vi "reward_behavior_michelle_visjitter_conswin.vi"() -> ()   [LabVIEW 2019]
doc: "The myRIO Project template acquires acceleration data from the onboard accelerometer and displays the changes of acceleration values in a waveform chart."
uses:
  <vilib>/Analysis/Matrix/Datatypes/RealMatrix.ctl
  <vilib>/myRIO/Common/Instrument Driver Framework/myRIO v1.0/Encoder/typedefs/Encoder Signal Mode.ctl
  <vilib>/myRIO/Instrument Drivers/Onboard IO/Encoder/typedefs/Encoder Reference.ctl
  <vilib>/myRIO/Common/Instrument Driver Framework/Utilities/typedefs/myRIO Generic Hardware Reference.ctl
  <vilib>/myRIO/Common/Instrument Driver Framework/Utilities/typedefs/Hardware Version Enum.ctl
  <vilib>/myRIO/Common/Instrument Driver Framework/Utilities/typedefs/myRIO v1.0 Reference.ctl
  <vilib>/myRIO/Common/Instrument Driver Framework/Utilities/typedefs/Generic FPGA Reference.ctl
  <vilib>/myRIO/Common/Instrument Driver Framework/myRIO v1.0/Encoder/typedefs/Encoder Channels Enum.ctl
  <vilib>/myRIO/Common/Instrument Driver Framework/myRIO v1.0/Encoder/typedefs/Encoder Configuration v1.0.ctl
  <vilib>/userdefined/High Color/nirio_resource_hc.ctl
  <vilib>/myRIO/Instrument Drivers/Onboard IO/DIO/typedefs/DIO Reference.ctl
  <vilib>/myRIO/Common/Instrument Driver Framework/myRIO v1.0/DIO/typedefs/DIO Channels List.ctl
  <vilib>/myRIO/Common/Instrument Driver Framework/myRIO v1.0/DIO/typedefs/DIO Channels Enum.ctl
  <vilib>/myRIO/Common/Instrument Driver Framework/Utilities/vis/Is FPGA Ref Available.vi
  <vilib>/myRIO/Common/Instrument Driver Framework/myRIO v1.0/Encoder/vis/myRIO v1.1 Open Encoder.vi
  <vilib>/myRIO/Instrument Drivers/Onboard IO/Encoder/vis/Read.vi
  <vilib>/myRIO/Common/Instrument Driver Framework/myRIO v1.0/DIO/vis/myRIO v1.1 Open DIO.vi
  <vilib>/myRIO/Instrument Drivers/Onboard IO/DIO/vis/Write.vi
  <vilib>/myRIO/Instrument Drivers/Onboard IO/DIO/vis/Read.vi
  <vilib>/myRIO/Common/Instrument Driver Framework/Utilities/vis/Validate Channels.vi
  <vilib>/myRIO/Common/Instrument Driver Framework/myRIO v1.0/Encoder/vis/myRIO v1.0 Reserve Encoder.vi
  <vilib>/myRIO/Common/Instrument Driver Framework/myRIO v1.0/DIO/vis/myRIO v1.0 Reserve DIO.vi
  <vilib>/myRIO/Common/Instrument Driver Framework/myRIO v1.0/Encoder/vis/myRIO v1.0 Build MUX Configuration Encoder.vi
  <vilib>/myRIO/Common/Instrument Driver Framework/myRIO v1.0/Resource Manager/vis/myRIO v1.0 Reserve Channel List.vi
  <vilib>/myRIO/Common/Instrument Driver Framework/myRIO v1.0/DIO/vis/myRIO v1.0 Build MUX Configuration DIO.vi
  <vilib>/myRIO/Common/Instrument Driver Framework/myRIO v1.0/Resource Manager/vis/myRIO v1.0 Create Configuration List.vi
  <vilib>/myRIO/Common/Instrument Driver Framework/myRIO v1.0/Resource Manager/vis/myRIO v1.0 Reserve Channel.vi
  <vilib>/myRIO/Common/Instrument Driver Framework/myRIO v1.0/Resource Manager/vis/myRIO v1.0 Unreserve Channel.vi
  <vilib>/myRIO/Common/Instrument Driver Framework/myRIO v1.0/Resource Manager/vis/myRIO v1.0 Build Mutex Name.vi
  <vilib>/Utility/VariantDataType/GetNumericInfo.vi
  <vilib>/Utility/error.llb/Error Cluster From Error Code.vi
  <vilib>/myRIO/Common/Instrument Driver Framework/myRIO v1.0/myRIO v1.1 Open.vi
  <vilib>/myRIO/Common/Instrument Driver Framework/Utilities/vis/IO Manager.vi
  <vilib>/myRIO/Common/Instrument Driver Framework/Utilities/vis/Configuration Manager.vi
  <vilib>/myRIO/Common/Instrument Driver Framework/myRIO v1.0/Resource Manager/vis/myRIO v1.0 Configure IO.vi
  <vilib>/myRIO/Common/Instrument Driver Framework/myRIO v1.0/myRIO v1.0 Close.vi
  <vilib>/myRIO/Common/Instrument Driver Framework/myRIO v1.0/Encoder/vis/myRIO v1.0 Configure Encoder.vi
  <vilib>/myRIO/Common/Instrument Driver Framework/myRIO v1.0/Encoder/vis/myRIO v1.0 Read Encoder.vi
  <vilib>/myRIO/Common/Instrument Driver Framework/myRIO v1.0/DIO/vis/myRIO v1.0 Read DIO.vi
  <vilib>/myRIO/Common/Instrument Driver Framework/myRIO v1.0/DIO/vis/myRIO v1.0 Write DIO.vi
  <vilib>/myRIO/Express VI/Onboard IO/Encoder/Encoder Express VI.xnode
  <vilib>/myRIO/Instrument Drivers/Onboard IO/Encoder/vis/myRIO Encoder Open.xnode
  <vilib>/myRIO/Express VI/Onboard IO/DI/DI Express VI.xnode
  <vilib>/myRIO/Instrument Drivers/Onboard IO/DIO/vis/myRIO DIO Open.xnode
  <vilib>/myRIO/Express VI/Onboard IO/DO/DO Express VI.xnode
  <vilib>/myRIO/Instrument Drivers/Onboard IO/Encoder/Encoder.lvlib
  <vilib>/myRIO/Instrument Drivers/Onboard IO/DIO/DIO.lvlib
  <vilib>/Analysis/Matrix/NI_Matrix.lvlib
panel:
  out "TimeOutDuration":i32
  out "ActiveTime":dbl
  out "ConsumptionGo":bool=TRUE
  out "Consumption_Period":i32
  out "Watch_Display":bool=TRUE
  in  "Give reward":bool
  out "Timings":dbl[](array[numeric])
  out "ISI":dbl
  out "ISI start time":dbl
  out "Time_out":bool=TRUE
  out "Time since lick":dbl
  out "Time of last lick":dbl
  out "Rewarded trials":dbl[](array[numeric])
  out "Rewards":u16
  out "Active Trial":bool
  out "Array temp2":T1
  out "Stimuli Loaded":bool
  out "Stim_ID":dbl[](array[numeric])
  out "Reward_mat":dbl[](array[numeric])
  out "Reward":bool=TRUE
  out "Frame clock":i32
  out "Licks":u32
  out "Lick":bool
  out "Time":dbl
  out "Stop":bool
  in  "Frames to collect":u32
  out "Overflow?":bool
  out "Counter Value":i32
  out "Velocity":dbl
  out "Velocity Plot":dbl[](graph)
  out "Velocity array":dbl[](array[numeric])
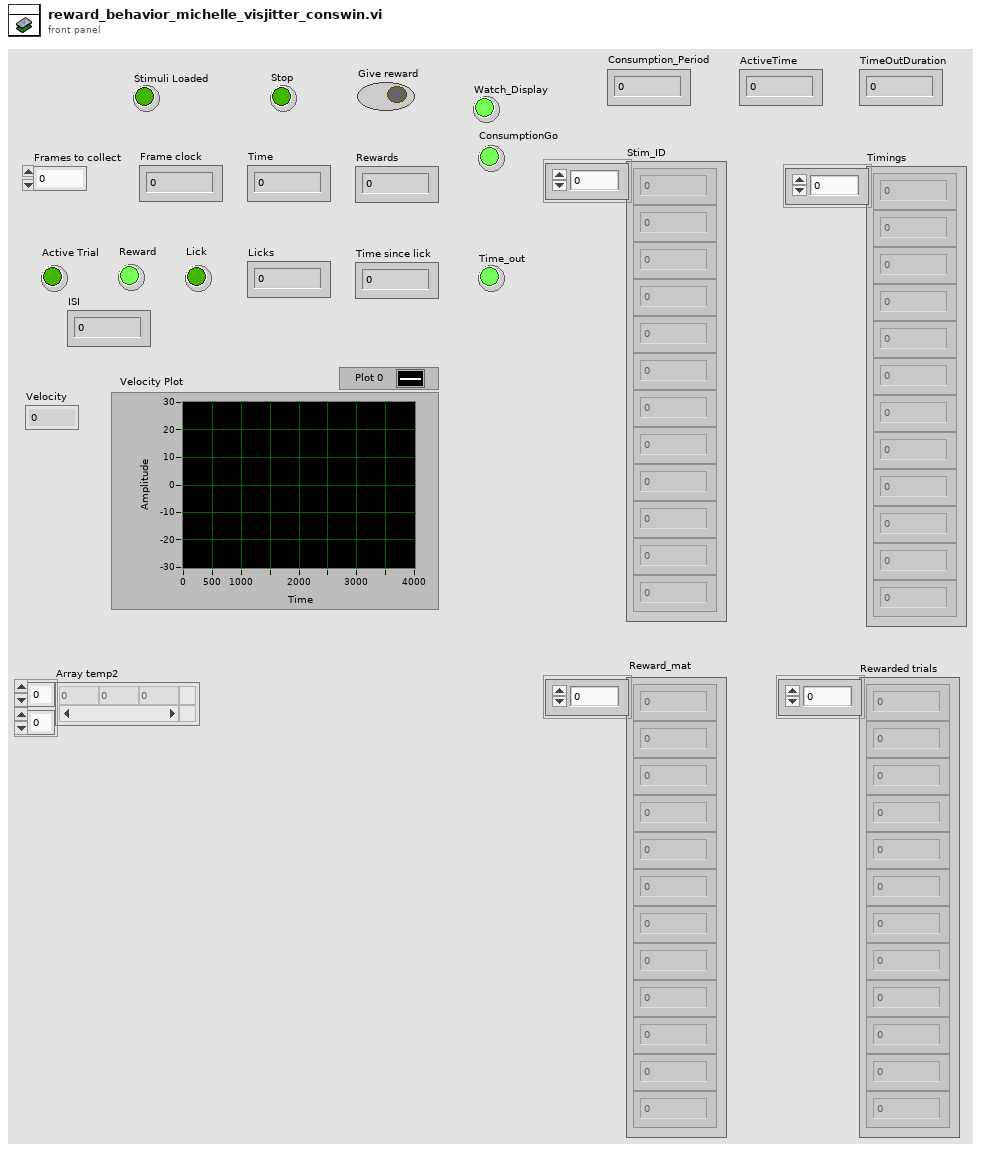
[diagram p1: front panel]
types:
  T1 = typedef "NI_Matrix.lvlib/RealMatrix.ctl" = dbl[][]
  T2 = typedef "Encoder.lvlib/Encoder Reference.ctl" = cluster{"myRIO Reference":T3, "Encoder Channels Enum":T7}
  T3 = typedef "myRIO Generic Hardware Reference.ctl" = cluster{"myRIO Model":T4, "myRIO Hardware Reference":T5}
  T4 = typedef "Hardware Version Enum.ctl" = enum16{"Unknown", "myRIO-1900", "myRIO-1950", "roboRIO", "NI ELVIS RIO CM", "ELVIS III"}
  T5 = typedef "myRIO v1.0 Reference.ctl" = cluster{"Generic FPGA Reference":T6, "Allow multiple opens":bool}
  T6 = typedef "Generic FPGA Reference.ctl" = refnum<k20>
  T7 = typedef "Encoder Channels Enum.ctl" = enum16{"Not Connected", "C/ENC0", "C/ENC1", "A/ENC", "A/ENC0", "A/ENC1", "A/ENC2", "A/ENC3", "A/ENC4", "A/ENC5", "A/ENC6", "A/ENC7", "A/ENC8", "A/ENC9", "B/ENC", "B/ENC0", "B/ENC1", "B/ENC2", "B/ENC3", "B/ENC4", "B/ENC5", "B/ENC6", "B/ENC7", "B/ENC8", "B/ENC9", "DIO/ENC0", "DIO/ENC1", "DIO/ENC2", "DIO/ENC3", "DIO/ENC4"}
  T8 = typedef "Encoder Signal Mode.ctl" = enum16{"Quadrature phase signal", "Step and direction signal"}
  T9 = typedef "nirio_resource_hc.ctl" = tag
  T10 = typedef "DIO.lvlib/DIO Reference.ctl" = cluster{"myRIO Reference":T3, "DIO Channels List":T11}
  T11 = typedef "DIO Channels List.ctl" = T12[]
  T12 = typedef "DIO Channels Enum.ctl" = enum16{"Not Connected", "C/DIO0", "C/DIO1", "C/DIO2", "C/DIO3", "C/DIO4", "C/DIO5", "C/DIO6", "C/DIO7", "A/DIO0", "A/DIO1", "A/DIO2", "A/DIO3", "A/DIO4", "A/DIO5", "A/DIO6", "A/DIO7", "A/DIO8", "A/DIO9", "A/DIO10", "A/DIO11", "A/DIO12", "A/DIO13", "A/DIO14", "A/DIO15", "A/DIO16", "A/DIO17", "A/DIO18", "A/DIO19", "B/DIO0", "B/DIO1", "B/DIO2", "B/DIO3", "B/DIO4", "B/DIO5", "B/DIO6", "B/DIO7", "B/DIO8", "B/DIO9", "B/DIO10", "B/DIO11", "B/DIO12", "B/DIO13", "B/DIO14", "B/DIO15", "B/DIO16", "B/DIO17", "B/DIO18", "B/DIO19", "LED0", "LED1", "LED2", "LED3", "Button0", "DIO/DIO0", "DIO/DIO1", "DIO/DIO2", "DIO/DIO3", "DIO/DIO4", "DIO/DIO5", "DIO/DIO6", "DIO/DIO7", "DIO/DIO8", "DIO/DIO9", "SPI/CS0", "SPI/CS1", "SPI/CS2", "SPI/CS3", "LED RADIO (Green)", "LED RADIO (Red)", "LED COMM (Green)", "LED COMM (Red)", "LED MODE (Green)", "LED MODE (Red)"}
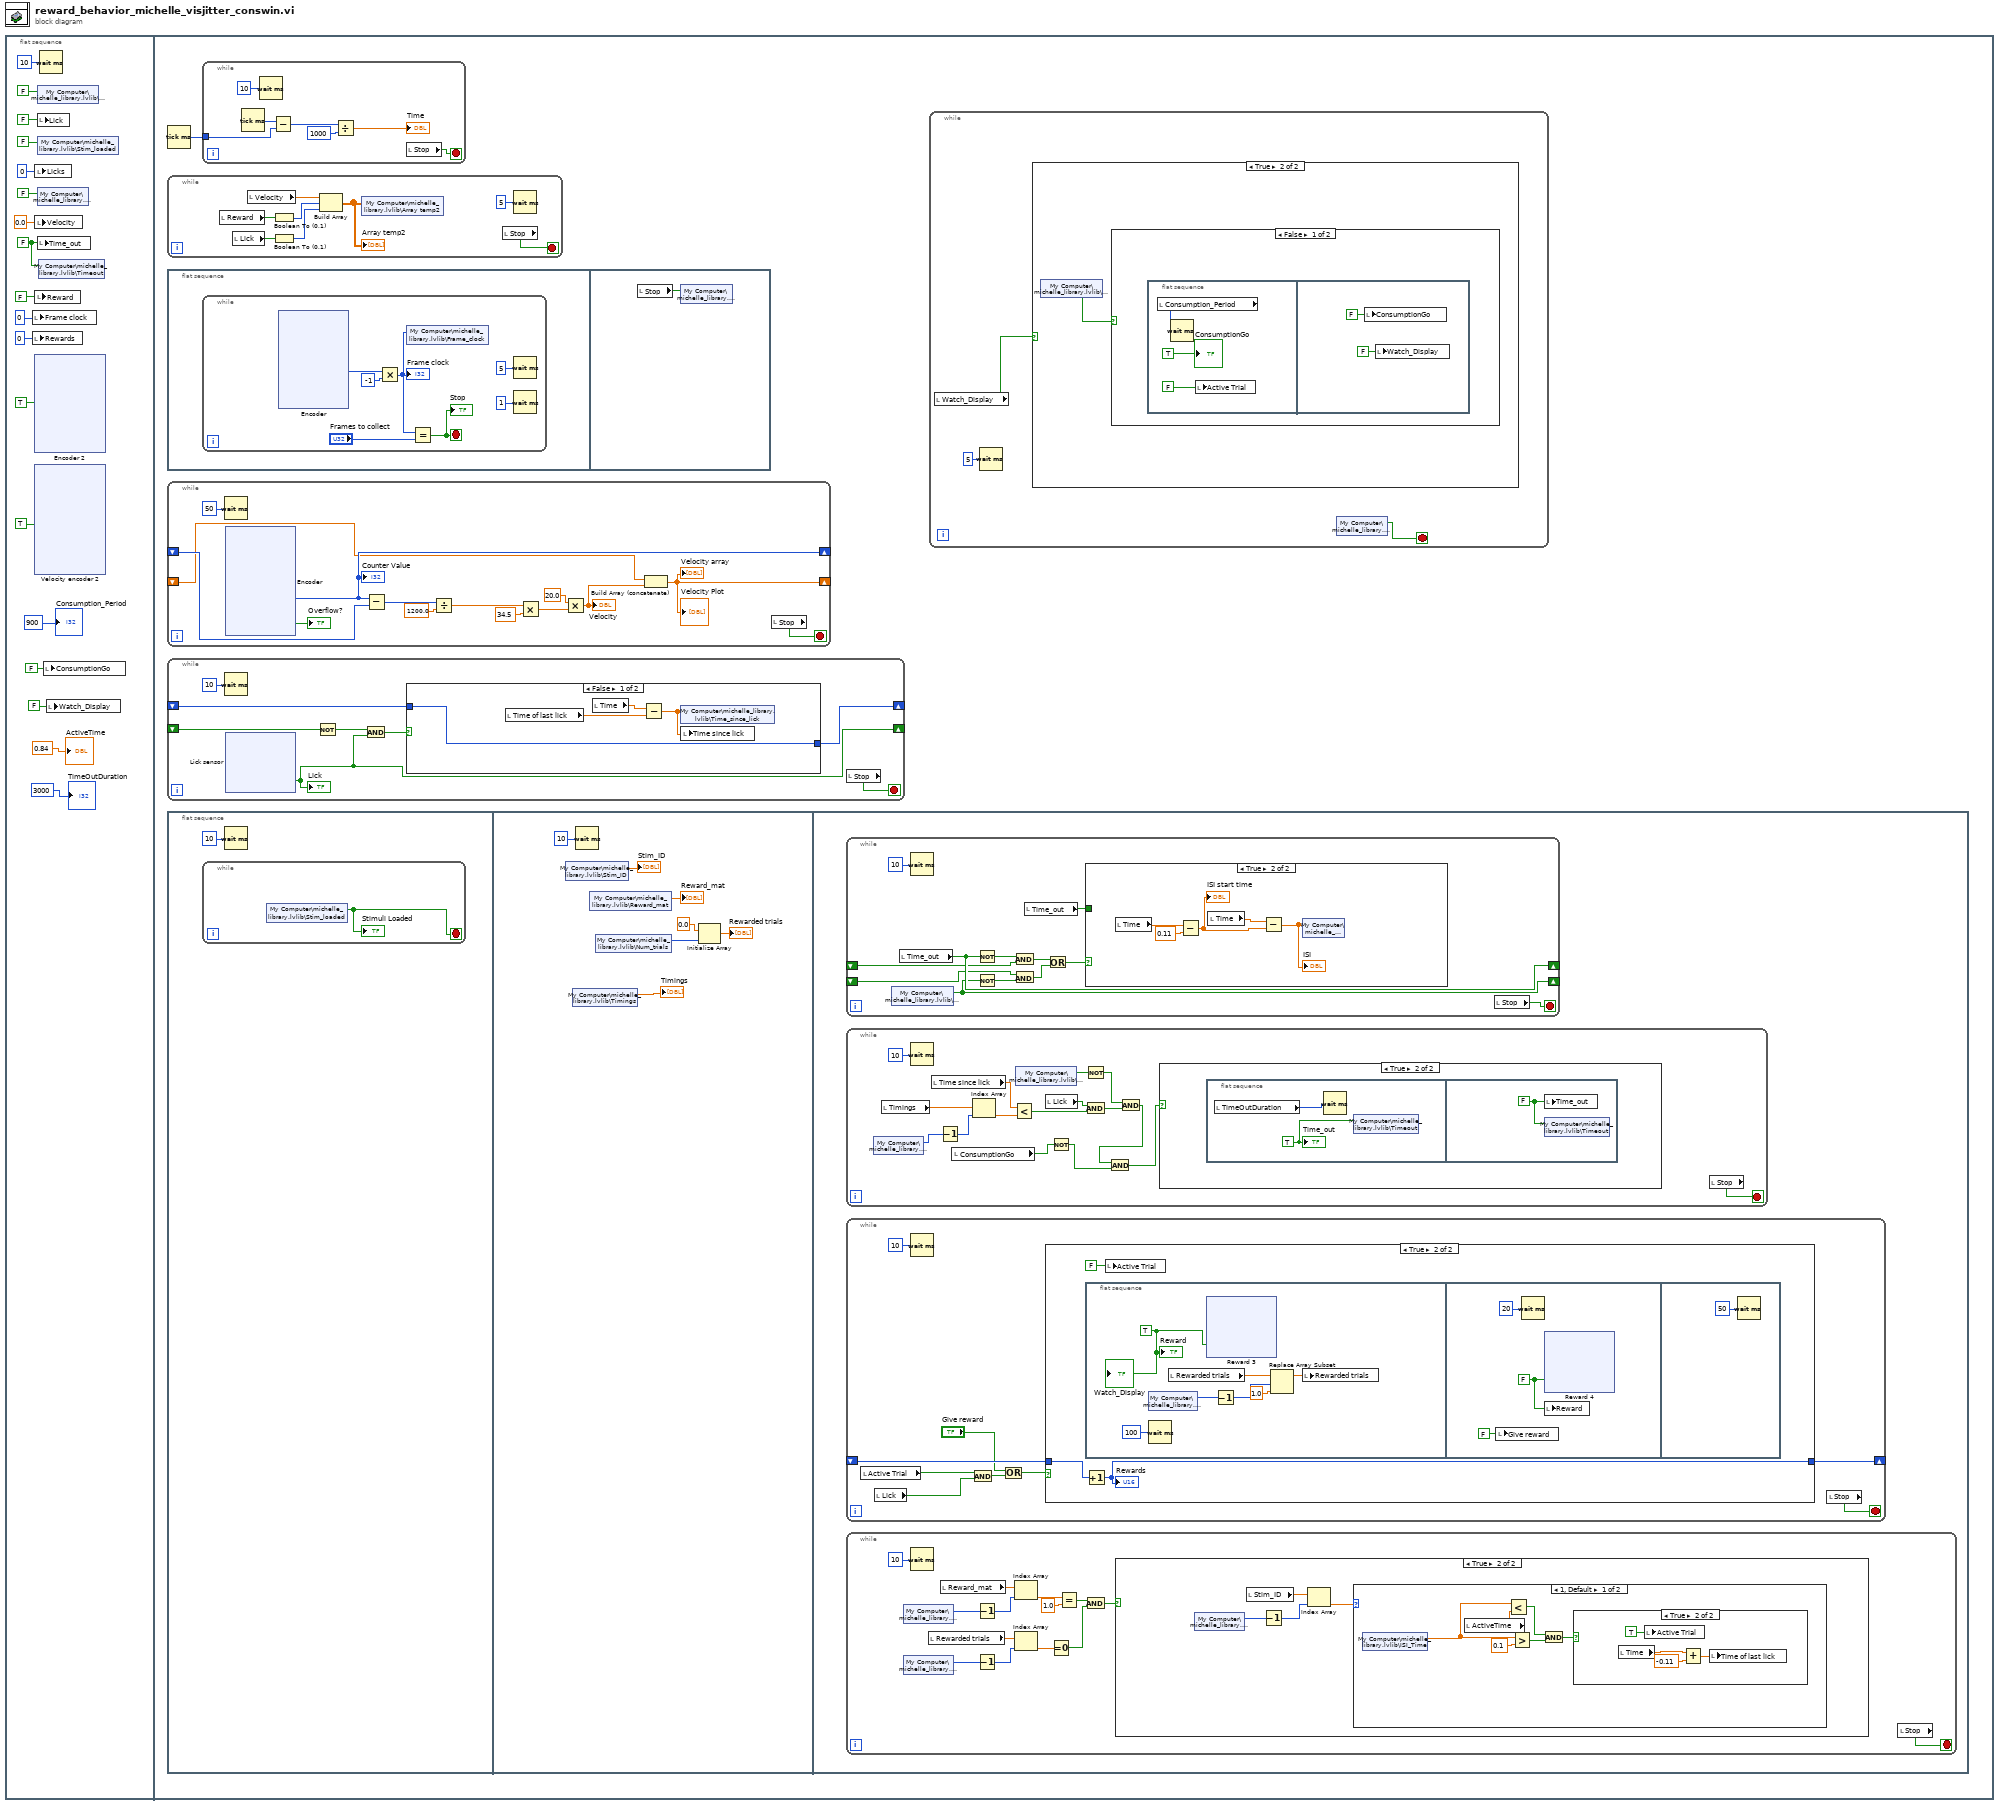
[diagram p0: block diagram]
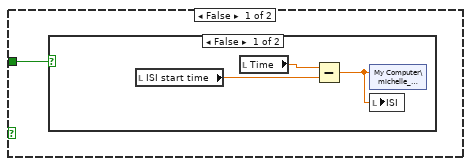
[diagram p5: hidden frame]
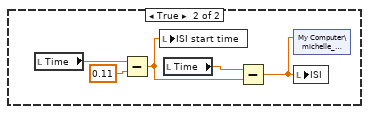
[diagram p6: hidden frame]
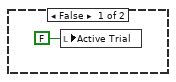
[diagram p7: hidden frame]
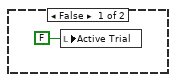
[diagram p8: hidden frame]
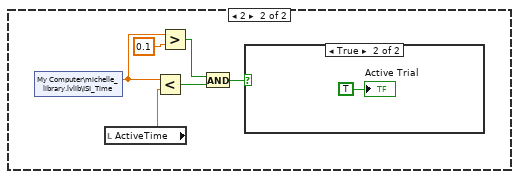
[diagram p9: hidden frame]
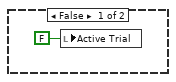
[diagram p10: hidden frame]
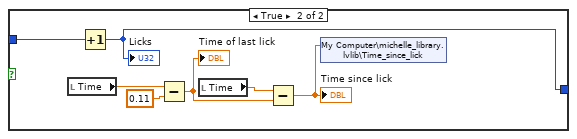
[diagram p12: hidden frame]
diagram:
  n1 = flat-sequence {
    frame #0 {
      w6 = FALSE ("Time_out")
      n2 = local write "Frame clock"(u32 0 ("Frames")) -> ()
      n3 = local write "Rewards"(u16 0 ("Rewards")) -> ()
      n4 = local write "Licks"(u32 0 ("Licks")) -> ()
      n5 = local write "Velocity"(0.0 ("Velocity")) -> ()
      n6 = local write "Reward"(FALSE ("Give reward")) -> ()
      n7 = xnode "Encoder 2"("Reset Counter"=TRUE) -> ()  [unwired: 1 in, 4 out]
      n8 = xnode "Velocity encoder 2"("Reset Counter"=TRUE) -> ()  [unwired: 1 in, 4 out]
      n9 = shared-variable "My Computer\\michelle_library.lvlib\\Display"(FALSE ("Display")) -> ()  [unwired: 1 in, 1 out]
      n10 = local write "Lick"(FALSE ("Lick")) -> ()
      n11 = shared-variable "My Computer\\michelle_library.lvlib\\Stim_loaded"(FALSE ("Stim_loaded")) -> ()  [unwired: 1 in, 1 out]
      n12 = shared-variable "My Computer\\michelle_library.lvlib\\Stop"(FALSE ("Stop")) -> ()  [unwired: 1 in, 1 out]
      n13 = local write "Time_out"(w6) -> ()
      n14 = shared-variable "My Computer\\michelle_library.lvlib\\Timeout"(w6) -> ()  [unwired: 1 in, 1 out]
      n15 = Wait (ms)(milliseconds to wait=u32 10) -> ()  [unwired: 1 out]
      n16 = local write "ConsumptionGo"(FALSE ("ConsumptionGo")) -> ()
      n17 = local write "Watch_Display"(FALSE ("Watch_Display")) -> ()
      "Consumption_Period" <- 900
      "ActiveTime" <- 0.84
      "TimeOutDuration" <- 3000
    }
    frame #1 {
      n18 = Tick Count (ms)() -> (millisecond timer value=w111:u32)
      n19 = while {
        stop <- w122 stop-if-true
        n20 = local read "Reward"() -> (w127:bool)
        n21 = local read "Lick"() -> (w128:bool)
        n22 = local read "Velocity"() -> (w126:dbl)
        n23 = Boolean To (0,1)(Boolean=w127) -> (0, 1=w125:i16)
        n24 = Boolean To (0,1)(Boolean=w128) -> (0, 1=w124:i16)
        n25 = Build Array(w126, w125, w124) -> (w121:T1)
        "Array temp2" <- w121
        n26 = shared-variable "My Computer\\michelle_library.lvlib\\Array temp2"(w121) -> ()  [unwired: 1 in, 1 out]
        n27 = local read "Stop"() -> (w122:bool)
        n28 = Wait (ms)(milliseconds to wait=u32 5) -> ()  [unwired: 1 out]
      }
      n29 = flat-sequence {
        frame #0 {
          n30 = while {
            stop <- w316 stop-if-true
            n31 = xnode "Encoder"() -> ("Counter Value"=w320:i32)  [unwired: 2 in, 3 out]
            n32 = Multiply(x=w320, y=-1) -> (x*y=w315:i32)
            "Frame clock" <- w315
            n33 = shared-variable "My Computer\\michelle_library.lvlib\\Frame_clock"(w315) -> ()  [unwired: 1 in, 1 out]
            n34 = Equal?(x=w315, y="Frames to collect") -> (x = y?=w316:bool)
            "Stop" <- w316
            n35 = Wait (ms)(milliseconds to wait=u32 5) -> ()  [unwired: 1 out]
            n36 = Wait (ms)(milliseconds to wait=u32 1) -> ()  [unwired: 1 out]
          }
        }
        frame #1 {
          n37 = local read "Stop"() -> (w368:bool)
          n38 = shared-variable "My Computer\\michelle_library.lvlib\\Stop"(w368) -> ()  [unwired: 1 in, 1 out]
        }
      }
      n39 = while {
        shift-right: [w433] -> _
        shift-left: _ -> [w434]
        shift-right: [w425] -> _
        shift-left: _ -> [w424]
        stop <- w423 stop-if-true
        n40 = Wait (ms)(milliseconds to wait=u32 50) -> ()  [unwired: 1 out]
        n41 = xnode "Encoder"() -> ("Counter Value"=w433:i32, "Overflow?"=→"Overflow?":bool)  [unwired: 2 in, 2 out]
        "Counter Value" <- w433
        n42 = Subtract(x=w433, y=w434) -> (x-y=w426:i32)
        n43 = Divide(x=w426, y=1200.0 ("600")) -> (x/y=w431:dbl)
        n44 = Multiply(x=w431, y=34.5) -> (x*y=w429:dbl)
        n45 = Multiply(x=20.0, y=w429) -> (x*y=w427:dbl)
        "Velocity" <- w427
        n46 = Build Array (concatenate)(w424, w427) -> (w425:dbl[])
        "Velocity Plot" <- w425
        "Velocity array" <- w425
        n47 = local read "Stop"() -> (w423:bool)
      }
      n48 = while {
        shift-right: [w375] -> _
        shift-left: _ -> [w374]
        shift-right: [w369] -> _
        shift-left: _ -> [w372]
        stop <- w373 stop-if-true
        n49 = Wait (ms)(milliseconds to wait=u32 10) -> ()  [unwired: 1 out]
        n50 = xnode "Lick sensor"() -> ("C/DIO1 (DIO1)"=w369:bool)  [unwired: 1 in, 1 out]
        "Lick" <- w369
        n51 = Not(x=w372) -> (.not. x?=w371:bool)
        n52 = And(x=w371, y=w369) -> (x .and. y?=w370:bool)
        n53 = case shown="False" w370 {
          tunnel: [w380 w387] -> w375
          tunnel: w374 -> [w380 w386]
          frame False {
            n54 = local read "Time of last lick"() -> (w378:dbl)
            n55 = local read "Time"() -> (w379:dbl)
            n56 = Subtract(x=w379, y=w378) -> (x-y=w377:dbl)
            n57 = shared-variable "My Computer\\michelle_library.lvlib\\Time_since_lick"(w377) -> ()  [unwired: 1 in, 1 out]
            n58 = local write "Time since lick"(w377) -> ()
          }
          frame True {
            n59 = local read "Time"() -> (w383:dbl)
            n60 = Increment(x=w386) -> (x+1=w387:u32)
            "Licks" <- w387
            n61 = Subtract(x=w383, y=0.11) -> (x-y=w381:dbl)
            "Time of last lick" <- w381
            n62 = local read "Time"() -> (w385:dbl)
            n63 = Subtract(x=w385, y=w381) -> (x-y=w384:dbl)
            "Time since lick" <- w384
            n64 = shared-variable "My Computer\\michelle_library.lvlib\\Time_since_lick"(w384) -> ()  [unwired: 1 in, 1 out]
          }
        }
        n65 = local read "Stop"() -> (w373:bool)
      }
      n66 = flat-sequence {
        frame #0 {
          n67 = while {
            stop <- w130 stop-if-true
            n68 = shared-variable "My Computer\\michelle_library.lvlib\\Stim_loaded"() -> (w130:bool)  [unwired: 1 in, 1 out]
            "Stimuli Loaded" <- w130
          }
          n69 = Wait (ms)(milliseconds to wait=u32 10) -> ()  [unwired: 1 out]
        }
        frame #1 {
          n70 = shared-variable "My Computer\\michelle_library.lvlib\\Stim_ID"() -> (→"Stim_ID":dbl[])  [unwired: 1 in, 1 out]
          n71 = shared-variable "My Computer\\michelle_library.lvlib\\Timings"() -> (→"Timings":dbl[])  [unwired: 1 in, 1 out]
          n72 = Wait (ms)(milliseconds to wait=u32 10) -> ()  [unwired: 1 out]
          n73 = shared-variable "My Computer\\michelle_library.lvlib\\Reward_mat"() -> (→"Reward_mat":dbl[])  [unwired: 1 in, 1 out]
          n74 = shared-variable "My Computer\\michelle_library.lvlib\\Num_trials"() -> (w134:u32)  [unwired: 1 in, 1 out]
          n75 = Initialize Array(0.0 ("element"), w134) -> (→"Rewarded trials":dbl[])
        }
        frame #2 {
          n76 = while {
            shift-right: [w167] -> _
            shift-left: _ -> [w165]
            shift-right: [w163] -> _
            shift-left: _ -> [w162]
            stop <- w168 stop-if-true
            n77 = shared-variable "My Computer\\michelle_library.lvlib\\Display"() -> (w163:bool)  [unwired: 1 in, 1 out]
            n78 = local read "Time_out"() -> (w167:bool)
            n79 = Wait (ms)(milliseconds to wait=u32 10) -> ()  [unwired: 1 out]
            n80 = Not(x=w167) -> (.not. x?=w166:bool)
            n81 = Not(x=w163) -> (.not. x?=w161:bool)
            n82 = And(x=w166, y=w165) -> (x .and. y?=w160:bool)
            n83 = And(x=w162, y=w161) -> (x .and. y?=w159:bool)
            n84 = local read "Time_out"() -> (w164:bool)
            n85 = Or(x=w160, y=w159) -> (x .or. y?=w158:bool)
            n86 = case shown="True" w158 {
              tunnel: w164 -> [w169 _]
              frame False {
                n87 = case shown="False" w169 {
                  frame False {
                    n88 = local read "ISI start time"() -> (w172:dbl)
                    n89 = local read "Time"() -> (w171:dbl)
                    n90 = Subtract(x=w171, y=w172) -> (x-y=w170:dbl)
                    n91 = shared-variable "My Computer\\michelle_library.lvlib\\ISI"(w170) -> ()  [unwired: 1 in, 1 out]
                    n92 = local write "ISI"(w170) -> ()
                  }
                  frame True {
                    n93 = local read "Time"() -> (w177:dbl)
                    n94 = Subtract(x=w177, y=0.11) -> (x-y=w174:dbl)
                    n95 = local write "ISI start time"(w174) -> ()
                    n96 = local read "Time"() -> (w175:dbl)
                    n97 = Subtract(x=w175, y=w174) -> (x-y=w173:dbl)
                    n98 = shared-variable "My Computer\\michelle_library.lvlib\\ISI"(w173) -> ()  [unwired: 1 in, 1 out]
                    n99 = local write "ISI"(w173) -> ()
                  }
                }
              }
              frame True {
                n100 = local read "Time"() -> (w182:dbl)
                n101 = Subtract(x=w182, y=0.11) -> (x-y=w179:dbl)
                "ISI start time" <- w179
                n102 = local read "Time"() -> (w180:dbl)
                n103 = Subtract(x=w180, y=w179) -> (x-y=w178:dbl)
                "ISI" <- w178
                n104 = shared-variable "My Computer\\michelle_library.lvlib\\ISI"(w178) -> ()  [unwired: 1 in, 1 out]
              }
            }
            n105 = local read "Stop"() -> (w168:bool)
          }
          n106 = while {
            stop <- w153 stop-if-true
            n107 = shared-variable "My Computer\\michelle_library.lvlib\\Trial"() -> (w143:u32)  [unwired: 1 in, 1 out]
            n108 = local read "Timings"() -> (w145:dbl[])
            n109 = Wait (ms)(milliseconds to wait=u32 10) -> ()  [unwired: 1 out]
            n110 = local read "Time since lick"() -> (w152:dbl)
            n111 = Decrement(x=w143) -> (x-1=w142:u32)
            n112 = local read "ConsumptionGo"() -> (w140:bool)
            n113 = Index Array(array=w145, index=w142) -> (element=w144:dbl)
            n114 = Less?(x=w152, y=w144) -> (x < y?=w151:bool)
            n115 = shared-variable "My Computer\\michelle_library.lvlib\\Display"() -> (w148:bool)  [unwired: 1 in, 1 out]
            n116 = local read "Lick"() -> (w150:bool)
            n117 = Not(x=w140) -> (.not. x?=w141:bool)
            n118 = Not(x=w148) -> (.not. x?=w147:bool)
            n119 = And(x=w150, y=w151) -> (x .and. y?=w146:bool)
            n120 = And(x=w147, y=w146) -> (x .and. y?=w139:bool)
            n121 = And(x=w139, y=w141) -> (x .and. y?=w138:bool)
            n122 = case shown="True" w138 {
              frame False {
              }
              frame True {
                n123 = flat-sequence {
                  frame #0 {
                    w155 = TRUE
                    n124 = local read "TimeOutDuration"() -> (w154:i32)
                    n125 = Wait (ms)(milliseconds to wait=w154) -> ()  [unwired: 1 out]
                    n126 = shared-variable "My Computer\\michelle_library.lvlib\\Timeout"(w155) -> ()  [unwired: 1 in, 1 out]
                    "Time_out" <- w155
                  }
                  frame #1 {
                    w156 = FALSE ("Timeout")
                    n127 = local write "Time_out"(w156) -> ()
                    n128 = shared-variable "My Computer\\michelle_library.lvlib\\Timeout"(w156) -> ()  [unwired: 1 in, 1 out]
                  }
                }
              }
            }
            n129 = local read "Stop"() -> (w153:bool)
          }
          n130 = while {
            shift-right: [w227] -> _
            shift-left: _ -> [w226]
            stop <- w229 stop-if-true
            n131 = local read "Active Trial"() -> (w224:bool)
            n132 = local read "Lick"() -> (w225:bool)
            n133 = Wait (ms)(milliseconds to wait=u32 10) -> ()  [unwired: 1 out]
            n134 = And(x=w224, y=w225) -> (x .and. y?=w223:bool)
            n135 = Or(x="Give reward", y=w223) -> (x .or. y?=w222:bool)
            n136 = case shown="True" w222 {
              tunnel: [w230 w233] -> w227
              tunnel: w226 -> [w230 w232]
              frame False {
              }
              frame True {
                n137 = Increment(x=w232) -> (x+1=w233:u16)
                "Rewards" <- w233
                n138 = flat-sequence {
                  frame #0 {
                    w239 = TRUE ("C/DIO0 (DIO0)")
                    n139 = shared-variable "My Computer\\michelle_library.lvlib\\Trial"() -> (w238:u32)  [unwired: 1 in, 1 out]
                    n140 = Wait (ms)(milliseconds to wait=u32 100) -> ()  [unwired: 1 out]
                    n141 = local read "Rewarded trials"() -> (w236:dbl[])
                    n142 = xnode "Reward 3"("C/DIO0 (DIO0)"=w239) -> ()  [unwired: 1 in, 1 out]
                    n143 = Decrement(x=w238) -> (x-1=w237:u32)
                    n144 = Replace Array Subset(array=w236, new element=1.0 ("new element/subarray"), index=w237) -> (w234:dbl[])
                    n145 = local write "Rewarded trials"(w234) -> ()
                    "Reward" <- w239
                    "Watch_Display" <- w239
                  }
                  frame #1 {
                    w278 = FALSE ("C/DIO0 (DIO0)")
                    n146 = local write "Give reward"(FALSE ("Give reward")) -> ()
                    n147 = Wait (ms)(milliseconds to wait=u32 20) -> ()  [unwired: 1 out]
                    n148 = xnode "Reward 4"("C/DIO0 (DIO0)"=w278) -> ()  [unwired: 1 in, 1 out]
                    n149 = local write "Reward"(w278) -> ()
                  }
                  frame #2 {
                    n150 = Wait (ms)(milliseconds to wait=u32 50) -> ()  [unwired: 1 out]
                  }
                }
                n151 = local write "Active Trial"(FALSE ("Active Trial")) -> ()
              }
            }
            n152 = local read "Stop"() -> (w229:bool)
          }
          n153 = while {
            stop <- w196 stop-if-true
            n154 = shared-variable "My Computer\\michelle_library.lvlib\\Trial"() -> (w192:u32)  [unwired: 1 in, 1 out]
            n155 = shared-variable "My Computer\\michelle_library.lvlib\\Trial"() -> (w188:u32)  [unwired: 1 in, 1 out]
            n156 = Wait (ms)(milliseconds to wait=u32 10) -> ()  [unwired: 1 out]
            n157 = local read "Rewarded trials"() -> (w189:dbl[])
            n158 = local read "Reward_mat"() -> (w191:dbl[])
            n159 = Decrement(x=w192) -> (x-1=w193:u32)
            n160 = Decrement(x=w188) -> (x-1=w187:u32)
            n161 = Index Array(array=w191, index=w193) -> (element=w194:dbl)
            n162 = Index Array(array=w189, index=w187) -> (element=w186:dbl)
            n163 = Equal To 0?(x=w186) -> (x = 0?=w185:bool)
            n164 = Equal?(x=w194, y=1.0) -> (x = y?=w184:bool)
            n165 = And(x=w184, y=w185) -> (x .and. y?=w183:bool)
            n166 = case shown="True" w183 {
              frame False {
                n167 = local write "Active Trial"(FALSE ("Active_trial")) -> ()
              }
              frame True {
                n168 = shared-variable "My Computer\\michelle_library.lvlib\\Trial"() -> (w199:u32)  [unwired: 1 in, 1 out]
                n169 = local read "Stim_ID"() -> (w201:dbl[])
                n170 = Decrement(x=w199) -> (x-1=w200:u32)
                n171 = Index Array(array=w201, index=w200) -> (element=w198:dbl)
                n172 = case shown="1, Default" w198 {
                  frame 1, Default {
                    n173 = shared-variable "My Computer\\michelle_library.lvlib\\ISI_Time"() -> (w207:dbl)  [unwired: 1 in, 1 out]
                    n174 = local read "ActiveTime"() -> (w202:dbl)
                    n175 = Less?(x=w207, y=w202) -> (x < y?=w205:bool)
                    n176 = Greater?(x=w207, y=0.1) -> (0:w204:bool)
                    n177 = And(x=w205, y=w204) -> (x .and. y?=w203:bool)
                    n178 = case shown="True" w203 {
                      frame False {
                        n179 = local write "Active Trial"(FALSE ("Active Trial")) -> ()
                      }
                      frame True {
                        n180 = local read "Time"() -> (w211:dbl)
                        n181 = local write "Active Trial"(TRUE ("Active Trial")) -> ()
                        n182 = Add(x=w211, y=-0.11) -> (x+y=w209:dbl)
                        n183 = local write "Time of last lick"(w209) -> ()
                      }
                    }
                  }
                  frame 2 {
                    n184 = shared-variable "My Computer\\michelle_library.lvlib\\ISI_Time"() -> (w217:dbl)  [unwired: 1 in, 1 out]
                    n185 = local read "ActiveTime"() -> (w213:dbl)
                    n186 = Less?(x=w217, y=w213) -> (x < y?=w215:bool)
                    n187 = Greater?(x=w217, y=0.1) -> (0:w216:bool)
                    n188 = And(x=w216, y=w215) -> (x .and. y?=w214:bool)
                    n189 = case shown="True" w214 {
                      frame False {
                        n190 = local write "Active Trial"(FALSE ("Active Trial")) -> ()
                      }
                      frame True {
                        "Active Trial" <- TRUE ("Active Trial")
                      }
                    }
                  }
                }
              }
            }
            n191 = local read "Stop"() -> (w196:bool)
          }
        }
      }
      n192 = while {
        tunnel: w111 -> [w488]
        stop <- w486 stop-if-true
        n193 = Tick Count (ms)() -> (millisecond timer value=w489:u32)
        n194 = Wait (ms)(milliseconds to wait=u32 10) -> ()  [unwired: 1 out]
        n195 = Subtract(x=w489, y=w488) -> (x-y=w485:u32)
        n196 = Divide(x=w485, y=u32 1000) -> (x/y=→"Time":dbl)
        n197 = local read "Stop"() -> (w486:bool)
      }
      n198 = while {
        stop <- w114 stop-if-true
        n199 = local read "Watch_Display"() -> (w113:bool)
        n200 = Wait (ms)(milliseconds to wait=u32 5) -> ()  [unwired: 1 out]
        n201 = case shown="True" w113 {
          frame False {
          }
          frame True {
            n202 = shared-variable "My Computer\\michelle_library.lvlib\\Display"() -> (w115:bool)  [unwired: 1 in, 1 out]
            n203 = case shown="False" w115 {
              frame False {
                n204 = flat-sequence {
                  frame #0 {
                    n205 = local read "Consumption_Period"() -> (w118:i32)
                    n206 = Wait (ms)(milliseconds to wait=w118) -> ()  [unwired: 1 out]
                    n207 = local write "Active Trial"(FALSE) -> ()
                    "ConsumptionGo" <- TRUE
                  }
                  frame #1 {
                    n208 = local write "ConsumptionGo"(FALSE ("ConsumptionGo")) -> ()
                    n209 = local write "Watch_Display"(FALSE ("Watch_Display")) -> ()
                  }
                }
              }
              frame True {
              }
            }
          }
        }
        n210 = shared-variable "My Computer\\michelle_library.lvlib\\Stop"() -> (w114:bool)  [unwired: 1 in, 1 out]
      }
    }
  }
